vi "PathLength.vi"(4 "PathIn":T1[](array[typedef])) -> (0 "Path Length":dbl, 1 "PathOut":T1[](array[typedef]), 2 "IndexedPathLength":dbl[](array[numeric]))   [LabVIEW 2017]
uses:
  TypeDefs/Point2D.ctl
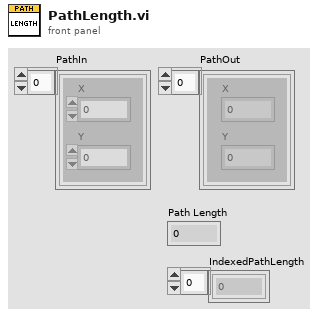
[diagram p1: front panel]
types:
  T1 = typedef "Point2D.ctl" = cluster{"X":dbl, "Y":dbl}
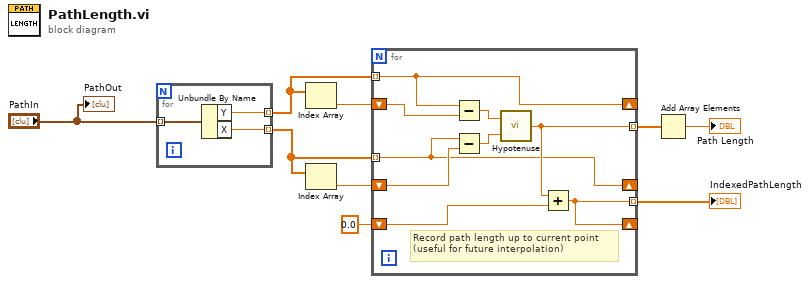
[diagram p0: block diagram]
diagram:
  n1 = for {
    tunnel: "PathIn" -> [w12] mode=indexing
    tunnel: [w11] -> w3 mode=indexing
    tunnel: [w10] -> w2 mode=indexing
    n2 = Unbundle By Name(w12) -> ("Y"=w11:dbl, "X"=w10:dbl)
  }
  n3 = Index Array(array=w3) -> (element=w8:dbl)  [unwired: 1 in]
  n4 = Index Array(array=w2) -> (element=w7:dbl)  [unwired: 1 in]
  n5 = for {
    tunnel: w3 -> [w21] mode=indexing
    tunnel: w2 -> [w13] mode=indexing
    shift-right: [w13] -> _
    shift-left: w7 -> [w14]
    shift-right: [w21] -> _
    shift-left: w8 -> [w20]
    tunnel: [w18] -> w6 mode=indexing
    shift-right: [w19] -> _
    shift-left: 0.0 -> [w17]
    tunnel: [w19] -> w4 mode=indexing
    # "Record path length up to current point\n(useful for future interpolation)"
    n6 = Subtract(x=w21, y=w20) -> (x-y=w16:dbl)
    n7 = Subtract(x=w13, y=w14) -> (x-y=w15:dbl)
    n8 = call "Hypotenuse.vi"("Y"=w15, "X"=w16) -> ("Hypotenuse"=w18:dbl)
    n9 = Add(x=w18, y=w17) -> (x+y=w19:dbl)
  }
  "IndexedPathLength" <- w4
  n10 = Add Array Elements(numeric array=w6) -> (sum=→"Path Length":dbl)
  "PathOut" <- "PathIn"
